vi "Print Number.vi"(8 "error in (no error)":errorcluster, 9 "Input":string, 11 "VISA resource name":refnum<visa-resource-name>) -> (0 "error out":errorcluster, 1 "Output":string, 3 "VISA resource name out":refnum<visa-resource-name>, 4 "Command String":string)   [LabVIEW 2018, in "Keithley 2600 Series.lvlib"]
doc: "This VI instructs the instrument to print the contents of the test script variable or value named by Input, to the instrument's output data queue. The returned data will be formatted according to the instrument format attributes.\n\nSee Also: format.data, format.asciiprecision, format.byteorder\n\n<b>Functions and Attributes Used</b>\nprintnumber()"
uses:
  Keithley 2600 Series.lvlib
  GlobalVariables.vi
panel:
  # "(c) 2008 Keithley Instruments, Inc.  ALL RIGHTS RESERVED."
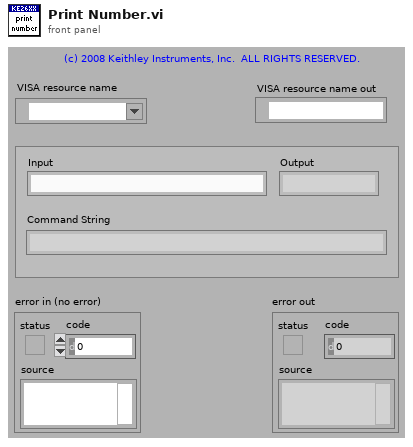
[diagram p1: front panel]
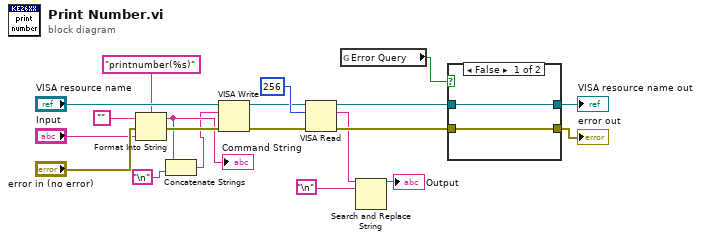
[diagram p0: block diagram]
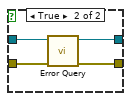
[diagram p2: hidden frame]
diagram:
  n1 = Format Into String(format string="printnumber(%s)" ("initial string"), initial string="", error in="error in (no error)", "Input") -> (resulting string=w5:string, error out=w17:errorcluster)
  "Command String" <- w5
  n2 = Concatenate Strings(w5, "\n") -> (w4:string)
  n3 = VISA Write(VISA resource name="VISA resource name", write buffer=w4, error in (no error)=w17) -> (VISA resource name out=w7:refnum<visa-resource-name>, error out=w8:errorcluster)  [unwired: 1 out]
  n4 = VISA Read(VISA resource name=w7, byte count=u32 256, error in (no error)=w8) -> (VISA resource name out=w13:refnum<visa-resource-name>, read buffer=w3:string, error out=w12:errorcluster)  [unwired: 1 out]
  n5 = global read "GlobalVariables.vi" "Error Query"() -> (w14:bool)
  n6 = Search and Replace String(input string=w3, search string="\n") -> (result string=→"Output":string)  [unwired: 6 in, 3 out]
  n7 = case shown="False" w14 {
    tunnel: w13 -> [w22 w26]
    tunnel: w12 -> [w21 w25]
    tunnel: [w22 w24] -> w11
    tunnel: [w21 w23] -> w20
    frame False {
    }
    frame True {
      n8 = call "Error Query.vi"("error in (no error)"=w25, "VISA resource name"=w26) -> ("error out"=w23:errorcluster, "VISA resource name out"=w24:refnum<visa-resource-name>)  [unwired: 8 out]
    }
  }
  "error out" <- w20
  "VISA resource name out" <- w11
